vi "Do That Thang.vi"(8 "error in (no error)":errorcluster, 9 "Lookup Table":refnum<data-value>, 11 "Popup in":refnum<class "Popup.lvclass">) -> (0 "error out":errorcluster, 3 "Popup out":refnum<class "Popup.lvclass">)   [LabVIEW 2017, in "Parallelizer Example.lvlib" / "Popup.lvclass"]
uses:
  <vilib>/gpm_packages/@cs/test-executive/Source/Sandbox/Parallelizer Example/Popup/Popup.lvclass
  C:/Program Files/National Instruments/LabVIEW 2017/vi.lib/ActorFramework/Actor/Actor.lvclass
  <vilib>/gpm_packages/@cs/lookup-table/Source/LookupTable/LookupTable.lvclass
  <vilib>/ActorFramework/Actor/Actor.lvclass/Actor.ctl
  <vilib>/ActorFramework/Message Enqueuer/Message Enqueuer.lvclass/Message Enqueuer.ctl
  <vilib>/gpm_packages/@cs/test-executive/Source/Sandbox/Parallelizer Example/Popup/Popup.lvclass/Popup.ctl
  <vilib>/ActorFramework/Message Enqueuer/Init from Existing Queue.vi
  <vilib>/ActorFramework/Message Enqueuer/Enqueue.vi
  <vilib>/ActorFramework/Stop Msg/Stop Msg.lvclass
  C:/Program Files/National Instruments/LabVIEW 2017/vi.lib/ActorFramework/Message/Message.lvclass
  <vilib>/ActorFramework/Message Priority Queue/Priority Enqueue.vi
  <vilib>/ActorFramework/Message Enqueuer/Message Enqueuer.lvclass
  <vilib>/ActorFramework/Actor/Actor.lvclass
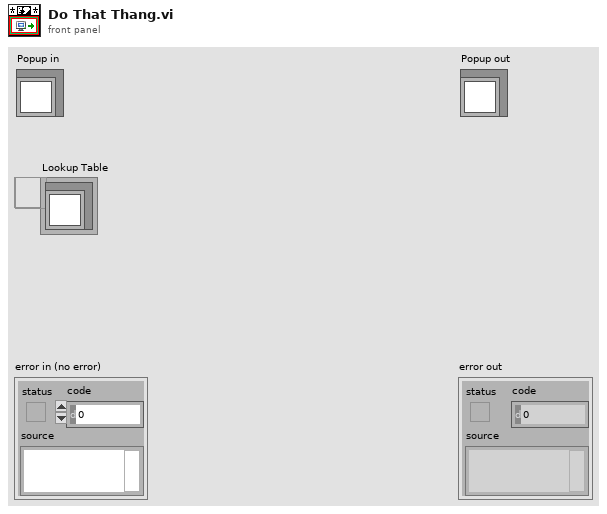
[diagram p1: front panel]
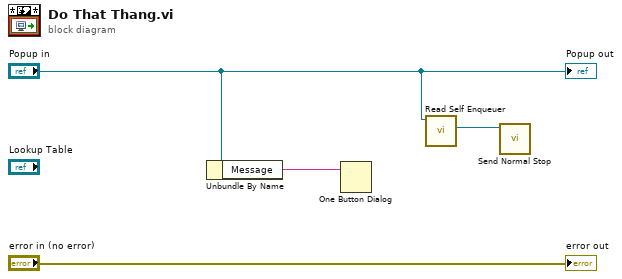
[diagram p0: block diagram]
diagram:
  n1 = Unbundle By Name("Popup in") -> ("Message"=w3:string)
  n2 = One Button Dialog(message=w3) -> ()  [unwired: 1 in, 1 out]
  n3 = call <vilib>:"Read Self Enqueuer.vi"("Actor"="Popup in") -> ("Self Enqueuer"=w1:refnum<class "Message Enqueuer.lvclass">)  [unwired: 10 in]
  n4 = call <vilib>:"Send Normal Stop.vi"("Message Enqueuer"=w1) -> ()  [unwired: 10 in, 1 out]
  "error out" <- "error in (no error)"
  "Popup out" <- "Popup in"
